vi "oa_Check Vector Data for Waveform Reference (1 Channel).vi"(0 "resampled signal":cluster{"r0":dbl, "dr":dbl, "Y":dbl[]}={"r0"=0.0, "dr"=1.0, "Y"=[]} {"r0" format="%.2p"; "dr" format="%.2p"; "Y" format="%.2f"}, 1 "reset? (True)":bool=TRUE, 5 "slow roll vectors":cdb[](array[numeric]) format="%.2f", 7 "orders to compensate":dbl[](array[numeric])=[1.0] format="%.2f", 11 "error out in":errorcluster) -> (2 "empty signal?":bool, 3 "parameter changed":bool, 4 "resampled signal dup":cluster{"r0":dbl, "dr":dbl, "Y":dbl[]}={"r0"=0.0, "dr"=1.0, "Y"=[]} {"r0" format="%.2p"; "dr" format="%.2p"; "Y" format="%.2f"}, 6 "slow roll vectors dup":cdb[](array[numeric]) format="%.2f", 8 "orders to compensate dup":dbl[](array[numeric])=[1.0] format="%.2f", 15 "error out":errorcluster)   [LabVIEW 2017, in "SoundVib_RefDataProcess.lvlib"]
uses:
  <vilib>/addons/Sound and Vibration/Order Analysis/Referece Data Processing/SoundVib_RefDataProcess.lvlib
  <vilib>/addons/Sound and Vibration/Order Analysis/Resample Order Tracking/SubVIs/OAT Verify Resampled Signal (Single Channel).vi
  <vilib>/addons/Sound and Vibration/Order Analysis/Resample Order Tracking/SoundVib_Resampling.lvlib
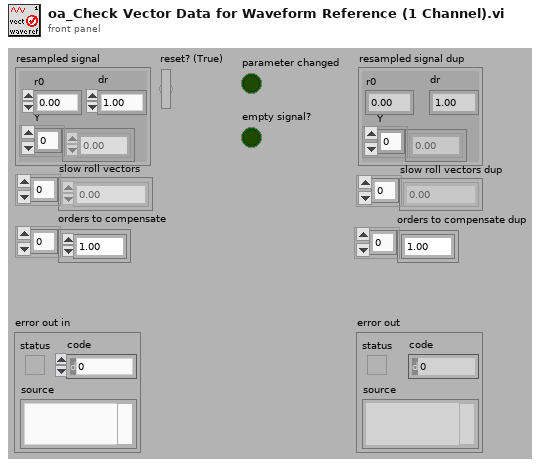
[diagram p1: front panel]
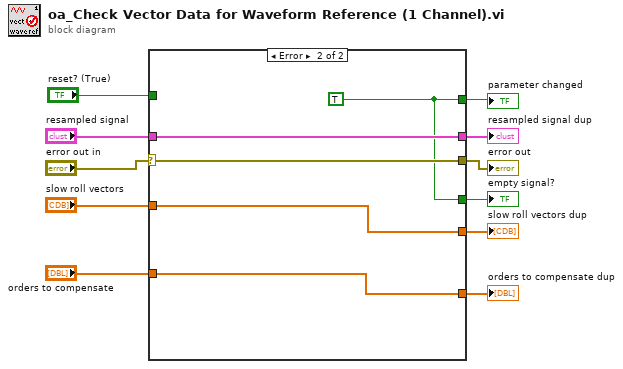
[diagram p0: block diagram]
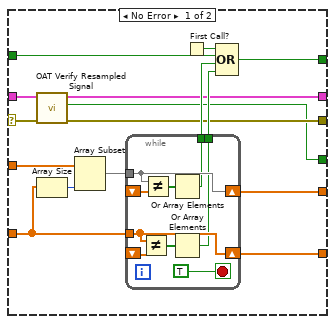
[diagram p2: hidden frame]
diagram:
  n1 = case shown="Error" "error out in" {
    selector: "error out in" -> [w18 w41]
    tunnel: [w17 w41] -> w10
    tunnel: [w19 w40] -> w8
    tunnel: "resampled signal" -> [w20 w40]
    tunnel: "slow roll vectors" -> [w16 w39]
    tunnel: "orders to compensate" -> [w13 w38]
    tunnel: [w27 w39] -> w5
    tunnel: [w26 w38] -> w4
    tunnel: "reset? (True)" -> [w25 _]
    tunnel: [w22 w37] -> w2
    tunnel: [w12 w37] -> w1
    frame No Error {
      n2 = call-poly <vilib>:"OAT Verify Resampled Signal.vi"("error in (no error)"=w18, "resampled signal"=w20) -> ("error out"=w17:errorcluster, "empty signal?"=w12:bool, "resampled signal dup"=w19:cluster{"r0":dbl, "dr":dbl, "Y":dbl[]})  [unwired: 7 in]
      n3 = Array Size(array=w13) -> (size(s)=w15:i32)
      n4 = Array Subset(array=w16, length=w15) -> (w14:cdb[])  [unwired: 1 in]
      n5 = while {
        tunnel: w14 -> [w34]
        tunnel: w13 -> [w31]
        shift-right: [w34] -> w27
        shift-left: _ -> [w35]
        shift-right: [w31] -> w26
        shift-left: _ -> [w32]
        tunnel: [w29] -> w24
        tunnel: [w28] -> w23
        stop <- TRUE stop-if-true
        n6 = Not Equal?(x=w31, y=w32) -> (x != y?=w30:bool[])
        n7 = Not Equal?(x=w34, y=w35) -> (x != y?=w33:bool[])
        n8 = Or Array Elements(Boolean array=w33) -> (logical OR=w29:bool)
        n9 = Or Array Elements(Boolean array=w30) -> (logical OR=w28:bool)
      }
      n10 = First Call?() -> (First Call?: T/F=w21:bool)
      n11 = Compound Arithmetic op=OR(w21, w25, w24, w23) -> (w22:bool)
    }
    frame Error {
      w37 = TRUE
    }
  }
  "resampled signal dup" <- w8
  "error out" <- w10
  "slow roll vectors dup" <- w5
  "orders to compensate dup" <- w4
  "parameter changed" <- w2
  "empty signal?" <- w1
